vi "Write Position.vi"(6 "DragOver Output":T2={"Displayed Row"=0, "Position"=enum."On Row", "Row's TreeItem index"=0, "indent"=0, "Accepted?"=FALSE, "Insertion index"=0, "Top left visible TreeItem index"=0, "Bar type"=enum."tilda up"}, 7 "Constant Sizes":T1, 8 "error in (no error)":errorcluster, 9 "Ref.Position":T5, 11 "BetterTreeBar in":refnum<class "BetterHorizontalBar.lvclass">) -> (0 "error out":errorcluster, 3 "BetterTreeBar out":refnum<class "BetterHorizontalBar.lvclass">)   [LabVIEW 2020, in "BetterDragAndDrop.lvlib" / "BetterHorizontalBar.lvclass"]
uses:
  BetterHorizontalBar.lvclass
  <vilib>/Utility/miscctls.llb/LVPositionTypeDef.ctl
  SubVIs/DragOver Output.ctl
  SubVIs/DragOverPosition.ctl
  SubVIs/Horizontal Bar Enumeration.ctl
  BetterHandle/Pixel Constants.ctl
  BetterHorizontalBar.lvclass/BetterHorizontalBar.ctl
  BetterHandle/BetterHandle.lvclass
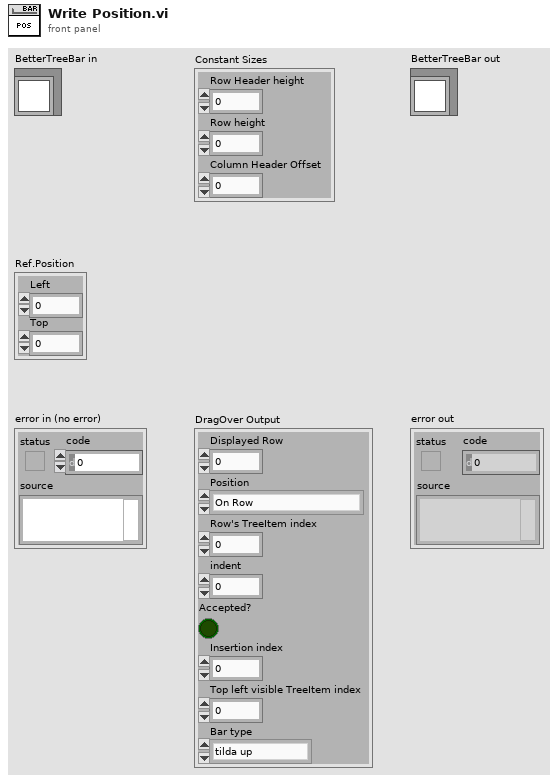
[diagram p1: front panel]
types:
  T1 = typedef "BetterDragAndDrop.lvlib/BetterHandle.lvclass/Pixel Constants.ctl" = cluster{"Row Header height":i32, "Row height":i32, "Column Header Offset":i32}
  T2 = typedef "BetterDragAndDrop.lvlib/BetterHandle.lvclass/DragOver Output.ctl" = cluster{"Displayed Row":i32, "Position":T3, "Row's TreeItem index":i32, "indent":i32, "Accepted?":bool, "Insertion index":i32, "Top left visible TreeItem index":i32, "Bar type":T4}
  T3 = typedef "BetterDragAndDrop.lvlib/BetterHandle.lvclass/DragOverPosition.ctl" = enum16{"On Row", "Inbetween"}
  T4 = typedef "BetterDragAndDrop.lvlib/BetterHorizontalBar.lvclass/Horizontal Bar Enumeration.ctl" = enum16{"None", "only bar", "tilda up"}
  T5 = typedef "LVPositionTypeDef.ctl" = cluster{"Left":i32, "Top":i32}
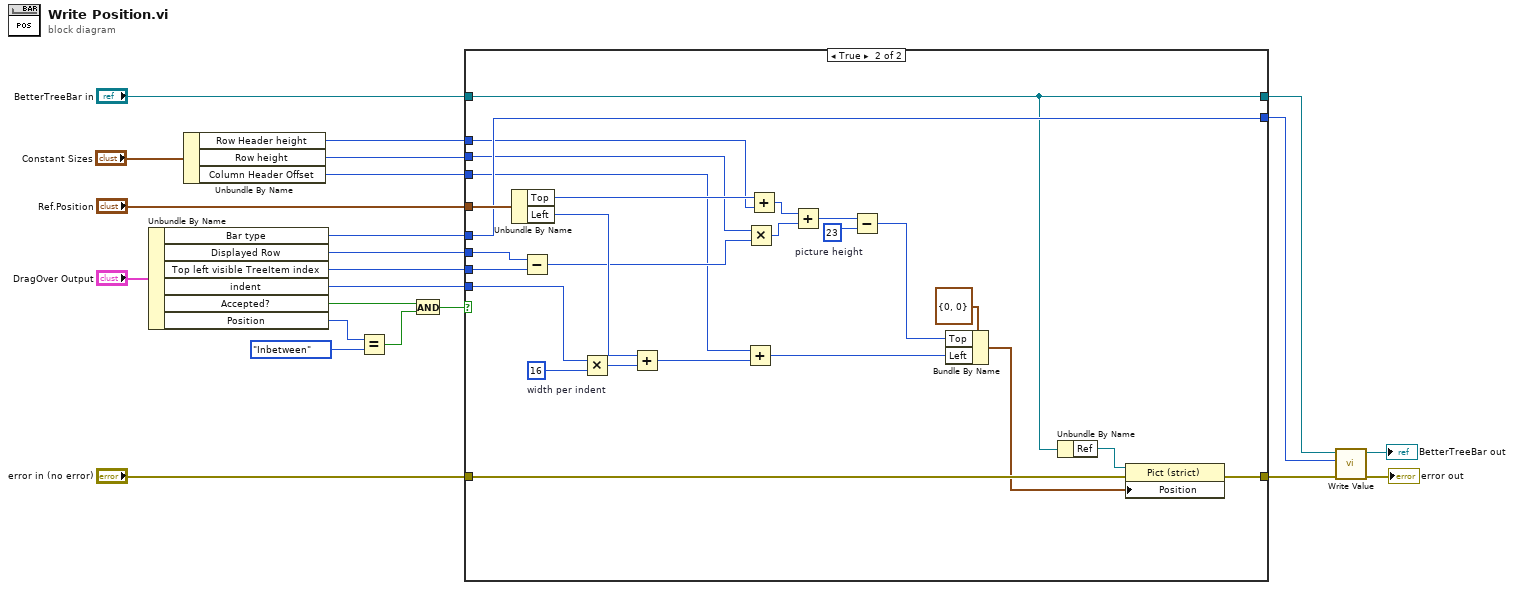
[diagram p0: block diagram]
diagram:
  n1 = Unbundle By Name("DragOver Output") -> ("Bar type"=w12:T4, "Displayed Row"=w13:i32, "Top left visible TreeItem index"=w20:i32, "indent"=w19:i32, "Accepted?"=w16:bool, "Position"=w17:T3)
  n2 = Unbundle By Name("Constant Sizes") -> ("Row Header height"=w3:i32, "Row height"=w2:i32, "Column Header Offset"=w1:i32)
  n3 = Equal?(x=w17, y=DragOverPosition."Inbetween") -> (x = y?=w15:bool)
  n4 = And(x=w16, y=w15) -> (x .and. y?=w14:bool)
  n5 = case shown="True" w14 {
    tunnel: w20 -> [_ w33]
    tunnel: "error in (no error)" -> [w24 w46]
    tunnel: [w24 w30] -> w8
    tunnel: "Ref.Position" -> [_ w45]
    tunnel: w19 -> [_ w41]
    tunnel: w13 -> [_ w34]
    tunnel: "BetterTreeBar in" -> [w23 w28]
    tunnel: [w23 w28] -> w9
    tunnel: w12 -> [_ w29]
    tunnel: [_ w29] -> w5
    tunnel: w3 -> [_ w27]
    tunnel: w2 -> [_ w26]
    tunnel: w1 -> [_ w25]
    frame False {
    }
    frame True {
      w38 = 16  # width per indent
      w47 = 23  # picture height
      n6 = Unbundle By Name(w45) -> ("Top"=w44:i32, "Left"=w39:i32)
      n7 = Subtract(x=w34, y=w33) -> (x-y=w32:i32)
      n8 = Multiply(x=w41, y=w38) -> (x*y=w40:i32)
      n9 = Add(x=w39, y=w40) -> (x+y=w37:i32)
      n10 = Add(x=w25, y=w37) -> (x+y=w36:i32)
      n11 = Multiply(x=w26, y=w32) -> (x*y=w50:i32)
      n12 = Add(x=w44, y=w27) -> (x+y=w49:i32)
      n13 = Add(x=w49, y=w50) -> (x+y=w48:i32)
      n14 = Subtract(x=w48, y=w47) -> (x-y=w35:i32)
      n15 = Bundle By Name(cluster=T5 {"Left"=0, "Top"=0} ("Position"), "Top"=w35, "Left"=w36) -> (w42:T5)
      n16 = Unbundle By Name(w28) -> ("Ref"=w31:refnum<vi>)
      n17 = property on="Property Node" class="Pict (strict)"(reference=w31, error in=w46, "Position"=w42) -> (error out=w30:errorcluster)  [unwired: 1 out]
    }
  }
  n18 = call "Write Value.vi"("error in (no error)"=w8, "New Value"=w5, "BetterTreeBar in"=w9) -> ("error out"=→"error out":errorcluster, "BetterTreeBar out"=→"BetterTreeBar out":refnum<class "BetterHorizontalBar.lvclass">)  [unwired: 7 in]
